vi "NMR_Long_RF_Pulse_Sequence.vi"() -> ()   [LabVIEW 2020]
uses:
  <instrlib>/niFgen/niFgen.llb/niFgen Waveform Type.ctl
  <instrlib>/niFgen/niFgen.llb/niFgen_ctl Trigger DigEdge - Edge Values (Ring).ctl
  <instrlib>/niFgen/niFgen.llb/niFgen_ctl Trigger Source Values (Ring).ctl
  <instrlib>/niFgen/niFgen.llb/niFgen Output Mode.ctl
  <instrlib>/niFgen/niFgen.llb/niFgen Trigger Mode.ctl
  <instrlib>/niFgen/niFgen.llb/niFgen Create Waveform (I16).vi
  <instrlib>/niFgen/niFgen.llb/niFgen Configure Digital Edge Start Trigger.vi
panel:
  in  "Frequency":dbl=1000000.0 format="%.4p"
  in  "Delay Time (ms)":u32=4000
  in  "Number of Scans":i32=16
  in  "DC Offset":dbl(knob) scale=-0.5..0.5 scale format="%#.1f"
  in  "Gain":dbl(knob)=1.3 min=0.0 max=5.0 scale=0.0..5.0 scale format="%#.1f"
  in  "FGEN Resource Name 2":refnum<k15>="FGEN1" caption="FGEN Resource Name"
  in  "Waveform Information Array":T1(array[cluster])=[{"Waveform Type"=7, "Amplitude"=0.0, "# of points"=1000}, {"Waveform Type"=7, "Amplitude"=1.0, "# of points"=1200}, {"Waveform Type"=7, "Amplitude"=0.0, "# of points"=255000}, {"Waveform Type"=7, "Amplitude"=1.0, "# of points"=2400}, {"Waveform Type"=7, "Amplitude"=0.0, "# of points"=500000}, {"Waveform Type"=7, "Amplitude"=1.0, "# of points"=2400}, {"Waveform Type"=7, "Amplitude"=0.0, "# of points"=500000}, {"Waveform Type"=7, "Amplitude"=1.0, "# of points"=2400}, {"Waveform Type"=7, "Amplitude"=0.0, "# of points"=500000}, {"Waveform Type"=7, "Amplitude"=1.0, "# of points"=2400}, {"Waveform Type"=7, "Amplitude"=0.0, "# of points"=500000}, {"Waveform Type"=7, "Amplitude"=1.0, "# of points"=2400}, {"Waveform Type"=7, "Amplitude"=0.0, "# of points"=500000}, {"Waveform Type"=7, "Amplitude"=1.0, "# of points"=2400}, {"Waveform Type"=7, "Amplitude"=0.0, "# of points"=500000}, {"Waveform Type"=7, "Amplitude"=1.0, "# of points"=2400}, {"Waveform Type"=7, "Amplitude"=0.0, "# of points"=500000}, {"Waveform Type"=7, "Amplitude"=1.0, "# of points"=2400}, {"Waveform Type"=7, "Amplitude"=0.0, "# of points"=500000}, {"Waveform Type"=7, "Amplitude"=1.0, "# of points"=2400}, {"Waveform Type"=7, "Amplitude"=0.0, "# of points"=500000}, {"Waveform Type"=7, "Amplitude"=1.0, "# of points"=2400}, {"Waveform Type"=7, "Amplitude"=0.0, "# of points"=500000}, {"Waveform Type"=7, "Amplitude"=1.0, "# of points"=2400}, {"Waveform Type"=7, "Amplitude"=0.0, "# of points"=500000}, {"Waveform Type"=7, "Amplitude"=1.0, "# of points"=2400}, {"Waveform Type"=7, "Amplitude"=0.0, "# of points"=500000}, {"Waveform Type"=7, "Amplitude"=1.0, "# of points"=2400}, {"Waveform Type"=7, "Amplitude"=0.0, "# of points"=500000}, {"Waveform Type"=7, "Amplitude"=1.0, "# of points"=2400}, {"Waveform Type"=7, "Amplitude"=0.0, "# of points"=500000}, {"Waveform Type"=7, "Amplitude"=1.0, "# of points"=2400}, {"Waveform Type"=7, "Amplitude"=0.0, "# of points"=500000}, {"Waveform Type"=7, "Amplitude"=1.0, "# of points"=2400}, {"Waveform Type"=7, "Amplitude"=0.0, "# of points"=500000}, {"Waveform Type"=7, "Amplitude"=1.0, "# of points"=2400}, {"Waveform Type"=7, "Amplitude"=0.0, "# of points"=500000}, {"Waveform Type"=7, "Amplitude"=1.0, "# of points"=2400}, {"Waveform Type"=7, "Amplitude"=0.0, "# of points"=500000}, {"Waveform Type"=7, "Amplitude"=1.0, "# of points"=2400}, {"Waveform Type"=7, "Amplitude"=0.0, "# of points"=500000}, {"Waveform Type"=7, "Amplitude"=1.0, "# of points"=2400}, {"Waveform Type"=7, "Amplitude"=0.0, "# of points"=500000}, {"Waveform Type"=7, "Amplitude"=1.0, "# of points"=2400}, {"Waveform Type"=7, "Amplitude"=0.0, "# of points"=500000}, {"Waveform Type"=7, "Amplitude"=1.0, "# of points"=2400}, {"Waveform Type"=7, "Amplitude"=0.0, "# of points"=500000}, {"Waveform Type"=7, "Amplitude"=1.0, "# of points"=2400}, {"Waveform Type"=7, "Amplitude"=0.0, "# of points"=500000}, {"Waveform Type"=7, "Amplitude"=1.0, "# of points"=2400}, {"Waveform Type"=7, "Amplitude"=0.0, "# of points"=500000}, {"Waveform Type"=7, "Amplitude"=1.0, "# of points"=2400}, {"Waveform Type"=7, "Amplitude"=0.0, "# of points"=500000}, {"Waveform Type"=7, "Amplitude"=1.0, "# of points"=2400}, {"Waveform Type"=7, "Amplitude"=0.0, "# of points"=500000}, {"Waveform Type"=7, "Amplitude"=1.0, "# of points"=2400}, {"Waveform Type"=7, "Amplitude"=0.0, "# of points"=500000}, {"Waveform Type"=7, "Amplitude"=1.0, "# of points"=2400}, {"Waveform Type"=7, "Amplitude"=0.0, "# of points"=500000}, {"Waveform Type"=7, "Amplitude"=1.0, "# of points"=2400}, {"Waveform Type"=7, "Amplitude"=0.0, "# of points"=500000}, {"Waveform Type"=7, "Amplitude"=1.0, "# of points"=2400}, {"Waveform Type"=7, "Amplitude"=0.0, "# of points"=500000}, {"Waveform Type"=7, "Amplitude"=1.0, "# of points"=2400}, {"Waveform Type"=7, "Amplitude"=0.0, "# of points"=500000}, {"Waveform Type"=7, "Amplitude"=1.0, "# of points"=2400}, {"Waveform Type"=7, "Amplitude"=0.0, "# of points"=500000}, {"Waveform Type"=7, "Amplitude"=1.0, "# of points"=2400}, {"Waveform Type"=7, "Amplitude"=0.0, "# of points"=500000}, {"Waveform Type"=7, "Amplitude"=1.0, "# of points"=2400}, {"Waveform Type"=7, "Amplitude"=0.0, "# of points"=500000}, {"Waveform Type"=7, "Amplitude"=1.0, "# of points"=2400}, {"Waveform Type"=7, "Amplitude"=0.0, "# of points"=500000}, {"Waveform Type"=7, "Amplitude"=1.0, "# of points"=2400}, {"Waveform Type"=7, "Amplitude"=0.0, "# of points"=500000}, {"Waveform Type"=7, "Amplitude"=1.0, "# of points"=2400}, {"Waveform Type"=7, "Amplitude"=0.0, "# of points"=500000}, {"Waveform Type"=7, "Amplitude"=1.0, "# of points"=2400}, {"Waveform Type"=7, "Amplitude"=0.0, "# of points"=500000}, {"Waveform Type"=7, "Amplitude"=1.0, "# of points"=2400}, {"Waveform Type"=7, "Amplitude"=0.0, "# of points"=500000}, {"Waveform Type"=7, "Amplitude"=1.0, "# of points"=2400}, {"Waveform Type"=7, "Amplitude"=0.0, "# of points"=500000}, {"Waveform Type"=7, "Amplitude"=1.0, "# of points"=2400}, {"Waveform Type"=7, "Amplitude"=0.0, "# of points"=500000}, {"Waveform Type"=7, "Amplitude"=1.0, "# of points"=2400}, {"Waveform Type"=7, "Amplitude"=0.0, "# of points"=500000}, {"Waveform Type"=7, "Amplitude"=1.0, "# of points"=2400}, {"Waveform Type"=7, "Amplitude"=0.0, "# of points"=500000}, {"Waveform Type"=7, "Amplitude"=1.0, "# of points"=2400}, {"Waveform Type"=7, "Amplitude"=0.0, "# of points"=500000}, {"Waveform Type"=7, "Amplitude"=1.0, "# of points"=2400}, {"Waveform Type"=7, "Amplitude"=0.0, "# of points"=500000}, {"Waveform Type"=7, "Amplitude"=1.0, "# of points"=2400}, {"Waveform Type"=7, "Amplitude"=0.0, "# of points"=500000}, {"Waveform Type"=7, "Amplitude"=1.0, "# of points"=2400}, {"Waveform Type"=7, "Amplitude"=0.0, "# of points"=500000}, {"Waveform Type"=7, "Amplitude"=1.0, "# of points"=2400}, {"Waveform Type"=7, "Amplitude"=0.0, "# of points"=500000}, {"Waveform Type"=7, "Amplitude"=1.0, "# of points"=2400}, {"Waveform Type"=7, "Amplitude"=0.0, "# of points"=500000}, {"Waveform Type"=7, "Amplitude"=1.0, "# of points"=2400}, {"Waveform Type"=7, "Amplitude"=0.0, "# of points"=500000}, {"Waveform Type"=7, "Amplitude"=1.0, "# of points"=2400}, {"Waveform Type"=7, "Amplitude"=0.0, "# of points"=500000}, {"Waveform Type"=7, "Amplitude"=1.0, "# of points"=2400}, {"Waveform Type"=7, "Amplitude"=0.0, "# of points"=500000}, {"Waveform Type"=7, "Amplitude"=1.0, "# of points"=2400}, {"Waveform Type"=7, "Amplitude"=0.0, "# of points"=500000}, {"Waveform Type"=7, "Amplitude"=1.0, "# of points"=2400}, {"Waveform Type"=7, "Amplitude"=0.0, "# of points"=500000}, {"Waveform Type"=7, "Amplitude"=1.0, "# of points"=2400}, {"Waveform Type"=7, "Amplitude"=0.0, "# of points"=500000}, {"Waveform Type"=7, "Amplitude"=1.0, "# of points"=2400}, {"Waveform Type"=7, "Amplitude"=0.0, "# of points"=500000}, {"Waveform Type"=7, "Amplitude"=1.0, "# of points"=2400}, {"Waveform Type"=7, "Amplitude"=0.0, "# of points"=500000}, {"Waveform Type"=7, "Amplitude"=1.0, "# of points"=2400}, {"Waveform Type"=7, "Amplitude"=0.0, "# of points"=500000}, {"Waveform Type"=7, "Amplitude"=1.0, "# of points"=2400}, {"Waveform Type"=7, "Amplitude"=0.0, "# of points"=500000}, {"Waveform Type"=7, "Amplitude"=1.0, "# of points"=2400}, {"Waveform Type"=7, "Amplitude"=0.0, "# of points"=500000}, {"Waveform Type"=7, "Amplitude"=1.0, "# of points"=2400}, {"Waveform Type"=7, "Amplitude"=0.0, "# of points"=500000}, {"Waveform Type"=7, "Amplitude"=1.0, "# of points"=2400}, {"Waveform Type"=7, "Amplitude"=0.0, "# of points"=500000}, {"Waveform Type"=7, "Amplitude"=1.0, "# of points"=2400}, {"Waveform Type"=7, "Amplitude"=0.0, "# of points"=500000}, {"Waveform Type"=7, "Amplitude"=1.0, "# of points"=2400}, {"Waveform Type"=7, "Amplitude"=0.0, "# of points"=500000}, {"Waveform Type"=7, "Amplitude"=1.0, "# of points"=2400}, {"Waveform Type"=7, "Amplitude"=0.0, "# of points"=500000}, {"Waveform Type"=7, "Amplitude"=1.0, "# of points"=2400}, {"Waveform Type"=7, "Amplitude"=0.0, "# of points"=500000}, {"Waveform Type"=7, "Amplitude"=1.0, "# of points"=2400}, {"Waveform Type"=7, "Amplitude"=0.0, "# of points"=500000}, {"Waveform Type"=7, "Amplitude"=1.0, "# of points"=2400}, {"Waveform Type"=7, "Amplitude"=0.0, "# of points"=500000}, {"Waveform Type"=7, "Amplitude"=1.0, "# of points"=2400}, {"Waveform Type"=7, "Amplitude"=0.0, "# of points"=500000}, {"Waveform Type"=7, "Amplitude"=1.0, "# of points"=2400}, {"Waveform Type"=7, "Amplitude"=0.0, "# of points"=500000}, {"Waveform Type"=7, "Amplitude"=1.0, "# of points"=2400}, {"Waveform Type"=7, "Amplitude"=0.0, "# of points"=500000}, {"Waveform Type"=7, "Amplitude"=1.0, "# of points"=2400}, {"Waveform Type"=7, "Amplitude"=0.0, "# of points"=500000}, {"Waveform Type"=7, "Amplitude"=1.0, "# of points"=2400}, {"Waveform Type"=7, "Amplitude"=0.0, "# of points"=500000}, {"Waveform Type"=7, "Amplitude"=1.0, "# of points"=2400}, {"Waveform Type"=7, "Amplitude"=0.0, "# of points"=500000}, {"Waveform Type"=7, "Amplitude"=1.0, "# of points"=2400}, {"Waveform Type"=7, "Amplitude"=0.0, "# of points"=500000}, {"Waveform Type"=7, "Amplitude"=1.0, "# of points"=2400}, {"Waveform Type"=7, "Amplitude"=0.0, "# of points"=500000}, {"Waveform Type"=7, "Amplitude"=1.0, "# of points"=2400}, {"Waveform Type"=7, "Amplitude"=0.0, "# of points"=500000}, {"Waveform Type"=7, "Amplitude"=1.0, "# of points"=2400}, {"Waveform Type"=7, "Amplitude"=0.0, "# of points"=500000}, {"Waveform Type"=7, "Amplitude"=1.0, "# of points"=2400}, {"Waveform Type"=7, "Amplitude"=0.0, "# of points"=500000}, {"Waveform Type"=7, "Amplitude"=1.0, "# of points"=2400}, {"Waveform Type"=7, "Amplitude"=0.0, "# of points"=500000}, {"Waveform Type"=7, "Amplitude"=1.0, "# of points"=2400}, {"Waveform Type"=7, "Amplitude"=0.0, "# of points"=500000}, {"Waveform Type"=7, "Amplitude"=1.0, "# of points"=2400}, {"Waveform Type"=7, "Amplitude"=0.0, "# of points"=500000}, {"Waveform Type"=7, "Amplitude"=1.0, "# of points"=2400}, {"Waveform Type"=7, "Amplitude"=0.0, "# of points"=500000}, {"Waveform Type"=7, "Amplitude"=1.0, "# of points"=2400}, {"Waveform Type"=7, "Amplitude"=0.0, "# of points"=500000}, {"Waveform Type"=7, "Amplitude"=1.0, "# of points"=2400}, {"Waveform Type"=7, "Amplitude"=0.0, "# of points"=500000}, {"Waveform Type"=7, "Amplitude"=1.0, "# of points"=2400}, {"Waveform Type"=7, "Amplitude"=0.0, "# of points"=500000}, {"Waveform Type"=7, "Amplitude"=1.0, "# of points"=2400}, {"Waveform Type"=7, "Amplitude"=0.0, "# of points"=500000}, {"Waveform Type"=7, "Amplitude"=1.0, "# of points"=2400}, {"Waveform Type"=7, "Amplitude"=0.0, "# of points"=500000}, {"Waveform Type"=7, "Amplitude"=1.0, "# of points"=2400}, {"Waveform Type"=7, "Amplitude"=0.0, "# of points"=500000}, {"Waveform Type"=7, "Amplitude"=1.0, "# of points"=2400}, {"Waveform Type"=7, "Amplitude"=0.0, "# of points"=500000}, {"Waveform Type"=7, "Amplitude"=1.0, "# of points"=2400}, {"Waveform Type"=7, "Amplitude"=0.0, "# of points"=500000}, {"Waveform Type"=7, "Amplitude"=1.0, "# of points"=2400}, {"Waveform Type"=7, "Amplitude"=0.0, "# of points"=500000}, {"Waveform Type"=7, "Amplitude"=1.0, "# of points"=2400}, {"Waveform Type"=7, "Amplitude"=0.0, "# of points"=500000}, {"Waveform Type"=7, "Amplitude"=1.0, "# of points"=2400}, {"Waveform Type"=7, "Amplitude"=0.0, "# of points"=500000}, {"Waveform Type"=7, "Amplitude"=1.0, "# of points"=2400}, {"Waveform Type"=7, "Amplitude"=0.0, "# of points"=500000}, {"Waveform Type"=7, "Amplitude"=1.0, "# of points"=2400}, {"Waveform Type"=7, "Amplitude"=0.0, "# of points"=500000}, {"Waveform Type"=7, "Amplitude"=1.0, "# of points"=2400}, {"Waveform Type"=7, "Amplitude"=0.0, "# of points"=500000}, {"Waveform Type"=7, "Amplitude"=1.0, "# of points"=2400}, {"Waveform Type"=7, "Amplitude"=0.0, "# of points"=500000}, {"Waveform Type"=7, "Amplitude"=1.0, "# of points"=2400}, {"Waveform Type"=7, "Amplitude"=0.0, "# of points"=10000000}] {"Amplitude" min=0.0 max=1.0 format="%.2f"; "Waveform Type" items=["Sine", "Cosine", "Triangle", "Square", "Sawtooth", "Increasing Ramp", "Decreasing Ramp", "DC Value"]}
  in  "Amplitude":dbl=0.35 format="%0_3g"
  in  "FGEN Resource Name":refnum<k15>="Dev1"
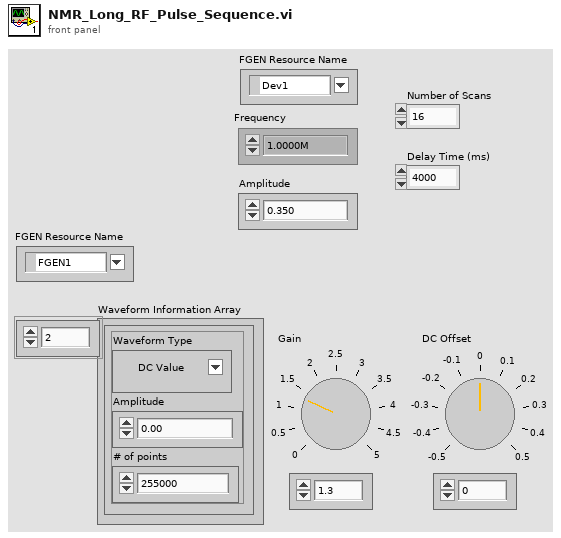
[diagram p1: front panel]
types:
  T1 = cluster{"Waveform Type":u16, "Amplitude":dbl, "# of points":u32}[]
  T2 = typedef "niFgen_ctl Trigger Source Values (Ring).ctl" = string
  T3 = typedef "niFgen Trigger Mode.ctl" = i32
  T4 = typedef "niFgen Output Mode.ctl" = u32
  T5 = typedef "niFgen_ctl Trigger DigEdge - Edge Values (Ring).ctl" = i32
  T6 = typedef "niFgen Waveform Type.ctl" = i32
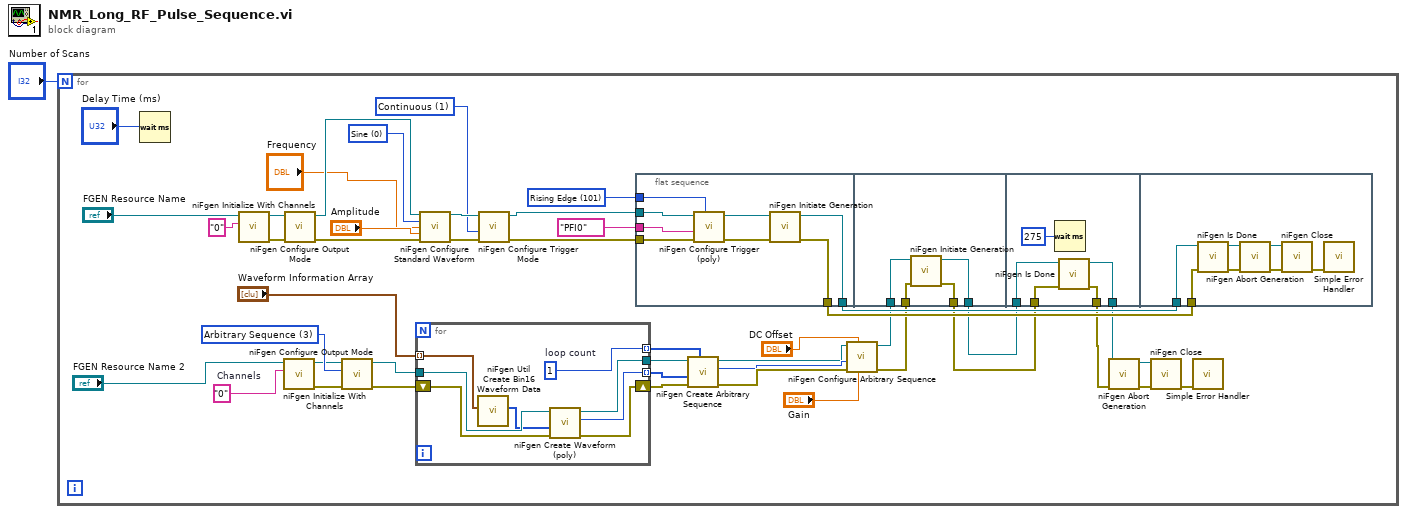
[diagram p0: block diagram]
diagram:
  n1 = for {
    N: "Number of Scans" -> [_]
    w8 = T3 1 items=["Single", "Continuous", "Stepped", "Burst"] ("Trigger Mode (default: 1=continuous)")
    w11 = "0"  # Channels
    w20 = T4 3 items=["Standard Function", "Frequency List", "Arbitrary Waveform", "Arbitrary Sequence", "Script"] ("output mode")
    w36 = T5 101 items=["Rising Edge"=101, "Falling Edge"=102] ("Edge (Rising)")
    w38 = T6 0 items=["Sine", "Square", "Triangle", "Ramp Up", "Ramp Down", "DC", "Noise", "User"] ("Waveform")
    n2 = Wait (ms)(milliseconds to wait="Delay Time (ms)") -> ()  [unwired: 1 out]
    n3 = call <instrlib>:"niFgen Initialize With Channels.vi"("Channel Name"="0", "Resource Name"="FGEN Resource Name") -> ("error out"=w43:errorcluster, "Instrument Handle Out"=w46:refnum<k15>)  [unwired: 8 in]
    n4 = call <instrlib>:"niFgen Initialize With Channels.vi"("Channel Name"=w11, "Resource Name"="FGEN Resource Name 2") -> ("error out"=w14:errorcluster, "Instrument Handle Out"=w13:refnum<k15>)  [unwired: 8 in]
    n5 = call <instrlib>:"niFgen Configure Output Mode.vi"("error in (no error)"=w43, "Instrument Handle"=w46) -> ("error out"=w42:errorcluster, "Instrument Handle Out"=w45:refnum<k15>)  [unwired: 7 in]
    n6 = call <instrlib>:"niFgen Configure Output Mode.vi"("error in (no error)"=w14, "Output Mode (default: 0=Standard Function)"=w20, "Instrument Handle"=w13) -> ("error out"=w24:errorcluster, "Instrument Handle Out"=w25:refnum<k15>)  [unwired: 6 in]
    n7 = for {
      shift-right: [w53] -> w21
      shift-left: w24 -> [w51]
      tunnel: [w54] -> w22
      tunnel: w25 -> [w52]
      tunnel: [w50] -> w23 mode=indexing
      tunnel: "Waveform Information Array" -> [w48] mode=indexing
      tunnel: [w47] -> w18 mode=indexing
      w47 = 1  # loop count
      n8 = call <instrlib>:"niFgen Util Create Bin16 Waveform Data.vi"("Waveform"=w48) -> ("Waveform Data"=w49:i16[])  [unwired: 10 in]
      n9 = call-poly <instrlib>:"niFgen Create Waveform (poly).vi"("error in (no error)"=w51, "Waveform Data Array"=w49, "Instrument Handle"=w52) -> ("error out"=w53:errorcluster, "Waveform Handle"=w50:i32, "Instrument Handle Out"=w54:refnum<k15>)  [unwired: 6 in]
    }
    n10 = call <instrlib>:"niFgen Configure Standard Waveform.vi"("Instrument Handle"=w45, "Waveform"=w38, "Frequency"="Frequency", "Amplitude"="Amplitude", "error in (no error)"=w42) -> ("Instrument Handle Out"=w44:refnum<k15>, "error out"=w41:errorcluster)  [unwired: 9 in]
    n11 = call <instrlib>:"niFgen Configure Trigger Mode.vi"("error in (no error)"=w41, "Trigger Mode (default: 1=continuous)"=w8, "Instrument Handle"=w44) -> ("error out"=w35:errorcluster, "Instrument Handle Out"=w33:refnum<k15>)  [unwired: 7 in]
    n12 = flat-sequence {
      tunnel: w36 -> [w61]
      tunnel: w35 -> [w60]
      tunnel: T2 "PFI0" ("Source") -> [w59]
      tunnel: w33 -> [w58]
      tunnel: [w57] -> w31
      tunnel: [w56] -> w32
      tunnel: w10 -> [w66]
      tunnel: w9 -> [w65]
      tunnel: [w64] -> w6
      tunnel: [w63] -> w5
      tunnel: w6 -> [w70]
      tunnel: w5 -> [w69]
      tunnel: [w68] -> w4
      tunnel: [w67] -> w3
      tunnel: w32 -> [w73]
      tunnel: w31 -> [w72]
      frame #0 {
        n13 = call-poly <instrlib>:"niFgen Configure Trigger (poly).vi"("Edge (Rising)"=w61, "error in (no error)"=w60, "Source"=w59, "Instrument Handle"=w58) -> ("error out"=w55:errorcluster, "Instrument Handle Out"=w62:refnum<k15>)  [unwired: 6 in]
        n14 = call <instrlib>:"niFgen Initiate Generation.vi"("error in (no error)"=w55, "Instrument Handle"=w62) -> ("error out"=w56:errorcluster, "Instrument Handle Out"=w57:refnum<k15>)  [unwired: 8 in]
      }
      frame #1 {
        n15 = call <instrlib>:"niFgen Initiate Generation.vi"("error in (no error)"=w66, "Instrument Handle"=w65) -> ("error out"=w64:errorcluster, "Instrument Handle Out"=w63:refnum<k15>)  [unwired: 8 in]
      }
      frame #2 {
        n16 = Wait (ms)(milliseconds to wait=u32 275) -> ()  [unwired: 1 out]
        n17 = call <instrlib>:"niFgen Is Done.vi"("error in (no error)"=w70, "Instrument Handle"=w69) -> ("error out"=w68:errorcluster, "Instrument Handle Out"=w67:refnum<k15>)  [unwired: 7 in, 1 out]
      }
      frame #3 {
        n18 = call <instrlib>:"niFgen Is Done.vi"("error in (no error)"=w73, "Instrument Handle"=w72) -> ("error out"=w76:errorcluster, "Instrument Handle Out"=w75:refnum<k15>)  [unwired: 7 in, 1 out]
        n19 = call <instrlib>:"niFgen Abort Generation.vi"("error in (no error)"=w76, "Instrument Handle"=w75) -> ("error out"=w77:errorcluster, "Instrument Handle Out"=w78:refnum<k15>)  [unwired: 8 in]
        n20 = call <instrlib>:"niFgen Close.vi"("error in (no error)"=w77, "Instrument Handle"=w78) -> ("error out"=w74:errorcluster)  [unwired: 9 in]
        n21 = call <vilib>:"Simple Error Handler.vi"("error in (no error)"=w74) -> ()  [unwired: 4 in, 5 out]
      }
    }
    n22 = call <instrlib>:"niFgen Create Arbitrary Sequence.vi"("Loop Counts Array"=w18, "error in (no error)"=w21, "Waveform Handles Array"=w23, "Instrument Handle"=w22) -> ("error out"=w28:errorcluster, "Sequence Handle"=w27:i32, "Instrument Handle Out"=w26:refnum<k15>)  [unwired: 5 in]
    n23 = call <instrlib>:"niFgen Configure Arbitrary Sequence.vi"("Gain"="Gain", "Offset"="DC Offset", "error in (no error)"=w28, "Sequence Handle"=w27, "Instrument Handle"=w26) -> ("error out"=w10:errorcluster, "Instrument Handle Out"=w9:refnum<k15>)  [unwired: 5 in]
    n24 = call <instrlib>:"niFgen Abort Generation.vi"("error in (no error)"=w4, "Instrument Handle"=w3) -> ("error out"=w29:errorcluster, "Instrument Handle Out"=w30:refnum<k15>)  [unwired: 8 in]
    n25 = call <instrlib>:"niFgen Close.vi"("error in (no error)"=w29, "Instrument Handle"=w30) -> ("error out"=w19:errorcluster)  [unwired: 9 in]
    n26 = call <vilib>:"Simple Error Handler.vi"("error in (no error)"=w19) -> ()  [unwired: 4 in, 5 out]
  }
